vi "pp2_log_SpawnRLLogger.vi"(10 "file path in":path, 11 "queue in":refnum<queue>) -> ()   [LabVIEW 2013]
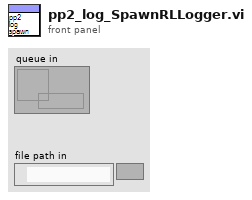
[diagram p1: front panel]
types:
  T1 = enum16{"open", "replace", "create", "open or create", "replace or create", "replace or create with confirmation"}
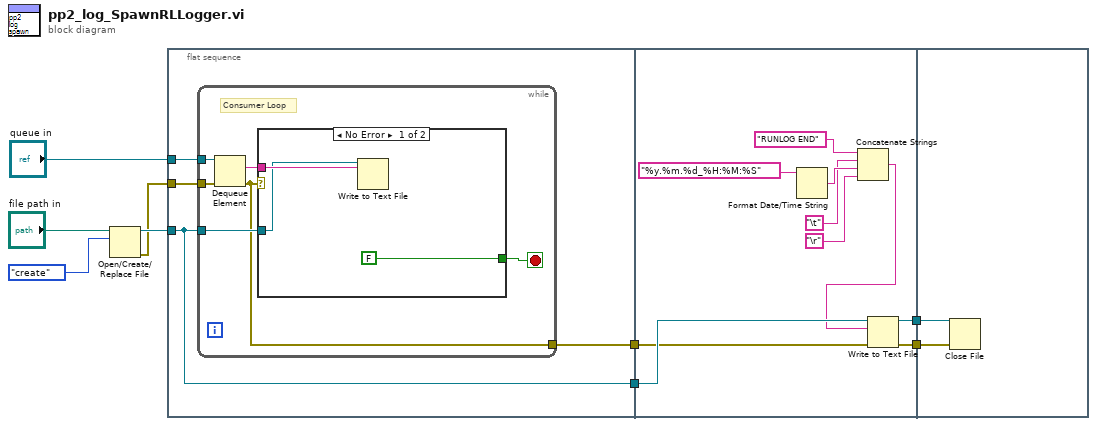
[diagram p0: block diagram]
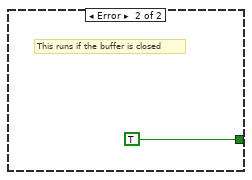
[diagram p2: hidden frame]
diagram:
  n1 = Open/Create/Replace File(file path (use dialog)="file path in", operation (0:open)=T1."create") -> (refnum out=w6:refnum<file>, error out=w3:errorcluster)  [unwired: 4 in, 1 out]
  n2 = flat-sequence {
    tunnel: "queue in" -> [w13]
    tunnel: w6 -> [w12]
    tunnel: [w12] -> w5
    tunnel: w3 -> [w11]
    tunnel: [w10] -> w2
    tunnel: w5 -> [w33]
    tunnel: [w26] -> w4
    tunnel: w2 -> [w25]
    tunnel: [w24] -> w1
    tunnel: w4 -> [w35]
    tunnel: w1 -> [w34]
    frame #0 {
      n3 = while {
        tunnel: w13 -> [w17]
        tunnel: w12 -> [w16]
        tunnel: w11 -> [w15]
        tunnel: [w14] -> w10
        stop <- w19 stop-if-true
        # "Consumer Loop"
        n4 = Dequeue Element(queue=w17, error in (no error)=w15) -> (element=w18:string, error out=w14:errorcluster)  [unwired: 1 in, 2 out]
        n5 = case shown="No Error" w14 {
          tunnel: [FALSE TRUE] -> w19
          tunnel: w18 -> [w21 _]
          tunnel: w16 -> [w20 _]
          frame No Error {
            n6 = Write to Text File(file (use dialog)=w20, text=w21) -> ()  [unwired: 2 in, 3 out]
          }
          frame Error {
            # "This runs if the buffer is closed"
          }
        }
      }
    }
    frame #1 {
      n7 = Format Date/Time String(time format string (%c)="%y.%m.%d_%H:%M:%S" ("pattern (all files)")) -> (date/time string=w32:string)  [unwired: 2 in]
      n8 = Concatenate Strings("RUNLOG END" ("string"), "\t", w32, "\r") -> (w27:string)
      n9 = Write to Text File(file (use dialog)=w33, text=w27, error in=w25) -> (refnum out=w26:refnum<file>, error out=w24:errorcluster)  [unwired: 1 in, 1 out]
    }
    frame #2 {
      n10 = Close File(refnum=w35, error in=w34) -> ()  [unwired: 2 out]
    }
  }
